vi "UNITEST MAIN v2.0.vi"() -> ()   [LabVIEW 2025] (continued)
        n1104 = call-poly "Enqueue Message.vi"("Priority Message? (F)"=TRUE, "Message"="Calculate Rotary", "Message Queue"=w1702) -> ("error out"=w1700:errorcluster, "dup Message Queue"=w1701:refnum<queue>)  [unwired: 7 in]
      }
      event "Clear List": Value Change {
        n1105 = event-data() -> ()  [unwired: 1 in, 1 out]
        n1106 = call-poly "Enqueue Message.vi"("Priority Message? (F)"=TRUE, "Message"="Clear List", "Message Queue"=w1707) -> ("error out"=w1705:errorcluster, "dup Message Queue"=w1706:refnum<queue>)  [unwired: 7 in]
      }
      event "Add to list": Value Change {
        n1107 = event-data() -> ()  [unwired: 1 in, 1 out]
        n1108 = call-poly "Enqueue Message.vi"("Priority Message? (F)"=TRUE, "Message"="Add to list", "Message Queue"=w1712) -> ("error out"=w1710:errorcluster, "dup Message Queue"=w1711:refnum<queue>)  [unwired: 7 in]
      }
      event "ClrLog": Value Change {
        n1109 = event-data() -> ()  [unwired: 1 in, 1 out]
        n1110 = call-poly "Enqueue Message.vi"("Priority Message? (F)"=TRUE, "Message"="ClrLog", "Message Queue"=w1717) -> ("error out"=w1715:errorcluster, "dup Message Queue"=w1716:refnum<queue>)  [unwired: 7 in]
      }
      event "Disable Axis Jog Soft Limits m": Value Change {
        n1111 = event-data() -> ()  [unwired: 1 in, 1 out]
        n1112 = call-poly "Enqueue Message.vi"("Priority Message? (F)"=TRUE, "Message"="Disable Axis Jog Soft Limits", "Message Queue"=w1722) -> ("error out"=w1720:errorcluster, "dup Message Queue"=w1721:refnum<queue>)  [unwired: 7 in]
      }
      event "Home Service": Value Change {
        n1113 = event-data() -> ()  [unwired: 1 in, 1 out]
        n1114 = call-poly "Enqueue Message.vi"("Priority Message? (F)"=TRUE, "Message"="Home Service", "Message Queue"=w1727) -> ("error out"=w1725:errorcluster, "dup Message Queue"=w1726:refnum<queue>)  [unwired: 7 in]
      }
      event "Edit Gain Constants": Value Change {
        n1115 = event-data() -> ()  [unwired: 1 in, 1 out]
        n1116 = call-poly "Enqueue Message.vi"("Priority Message? (F)"=TRUE, "Message"="Edit Gain Constants", "Message Queue"=w1732) -> ("error out"=w1730:errorcluster, "dup Message Queue"=w1731:refnum<queue>)  [unwired: 7 in]
      }
      event "Advanced Setting": Value Change {
        n1117 = event-data() -> ()  [unwired: 1 in, 1 out]
        n1118 = call-poly "Enqueue Message.vi"("Priority Message? (F)"=TRUE, "Message"="Advanced Setting", "Message Queue"=w1737) -> ("error out"=w1735:errorcluster, "dup Message Queue"=w1736:refnum<queue>)  [unwired: 7 in]
      }
      event "Password": Value Change {
        n1119 = event-data() -> ()  [unwired: 1 in, 1 out]
        n1120 = call-poly "Enqueue Message.vi"("Priority Message? (F)"=TRUE, "Message"="Password", "Message Queue"=w1742) -> ("error out"=w1740:errorcluster, "dup Message Queue"=w1741:refnum<queue>)  [unwired: 7 in]
      }
      event "Service About": Value Change {
        n1121 = event-data() -> ()  [unwired: 1 in, 1 out]
        n1122 = call-poly "Enqueue Message.vi"("Priority Message? (F)"=TRUE, "Message"="Service About", "Message Queue"=w1747) -> ("error out"=w1745:errorcluster, "dup Message Queue"=w1746:refnum<queue>)  [unwired: 7 in]
      }
      event "OPEN 1": Value Change {
        n1123 = event-data() -> ()  [unwired: 1 in, 1 out]
        n1124 = call-poly "Enqueue Message.vi"("Priority Message? (F)"=TRUE, "Message"="OPEN 1", "Message Queue"=w1752) -> ("error out"=w1750:errorcluster, "dup Message Queue"=w1751:refnum<queue>)  [unwired: 7 in]
      }
      event "OPEN 2": Value Change {
        n1125 = event-data() -> ()  [unwired: 1 in, 1 out]
        n1126 = call-poly "Enqueue Message.vi"("Priority Message? (F)"=TRUE, "Message"="OPEN 2", "Message Queue"=w1757) -> ("error out"=w1755:errorcluster, "dup Message Queue"=w1756:refnum<queue>)  [unwired: 7 in]
      }
      event "OPEN 3": Value Change {
        n1127 = event-data() -> ()  [unwired: 1 in, 1 out]
        n1128 = call-poly "Enqueue Message.vi"("Priority Message? (F)"=TRUE, "Message"="OPEN 3", "Message Queue"=w1762) -> ("error out"=w1760:errorcluster, "dup Message Queue"=w1761:refnum<queue>)  [unwired: 7 in]
      }
      event "OPEN 4": Value Change {
        n1129 = event-data() -> ()  [unwired: 1 in, 1 out]
        n1130 = call-poly "Enqueue Message.vi"("Priority Message? (F)"=TRUE, "Message"="OPEN 4", "Message Queue"=w1767) -> ("error out"=w1765:errorcluster, "dup Message Queue"=w1766:refnum<queue>)  [unwired: 7 in]
      }
      event "Refresh 2": Value Change {
        n1131 = event-data() -> ()  [unwired: 1 in, 1 out]
        n1132 = call-poly "Enqueue Message.vi"("Priority Message? (F)"=TRUE, "Message"="Refresh 2", "Message Queue"=w1772) -> ("error out"=w1770:errorcluster, "dup Message Queue"=w1771:refnum<queue>)  [unwired: 7 in]
      }
      event "Analysis Home new": Value Change {
        n1133 = event-data() -> ()  [unwired: 1 in, 1 out]
        n1134 = call-poly "Enqueue Message.vi"("Priority Message? (F)"=TRUE, "Message"="Analysis Home", "Message Queue"=w1777) -> ("error out"=w1775:errorcluster, "dup Message Queue"=w1776:refnum<queue>)  [unwired: 7 in]
      }
      event "Post Analysis": Value Change {
        n1135 = event-data() -> ()  [unwired: 1 in, 1 out]
        n1136 = call-poly "Enqueue Message.vi"("Priority Message? (F)"=TRUE, "Message"="Post Analysis", "Message Queue"=w1782) -> ("error out"=w1780:errorcluster, "dup Message Queue"=w1781:refnum<queue>)  [unwired: 7 in]
      }
      event "Scratch Mode": Value Change {
        n1137 = event-data() -> ()  [unwired: 1 in, 1 out]
        n1138 = call-poly "Enqueue Message.vi"("Priority Message? (F)"=TRUE, "Message"="Scratch Mode", "Message Queue"=w1787) -> ("error out"=w1785:errorcluster, "dup Message Queue"=w1786:refnum<queue>)  [unwired: 7 in]
      }
      event "Export": Value Change {
        n1139 = event-data() -> ()  [unwired: 1 in, 1 out]
        n1140 = call-poly "Enqueue Message.vi"("Priority Message? (F)"=TRUE, "Message"="Export", "Message Queue"=w1792) -> ("error out"=w1790:errorcluster, "dup Message Queue"=w1791:refnum<queue>)  [unwired: 7 in]
      }
      event "Traction Receipe Update Details": Value Change {
        n1141 = event-data() -> ()  [unwired: 1 in, 1 out]
        n1142 = call-poly "Enqueue Message.vi"("Priority Message? (F)"=TRUE, "Message"="Traction Receipe Update Details", "Message Queue"=w1797) -> ("error out"=w1795:errorcluster, "dup Message Queue"=w1796:refnum<queue>)  [unwired: 7 in]
      }
      event "Manual Write TRACTION": Value Change {
        n1143 = event-data() -> ()  [unwired: 1 in, 1 out]
        n1144 = call-poly "Enqueue Message.vi"("Priority Message? (F)"=TRUE, "Message"="Manual Write TRACTION", "Message Queue"=w1802) -> ("error out"=w1800:errorcluster, "dup Message Queue"=w1801:refnum<queue>)  [unwired: 7 in]
      }
      event "Manual Write Acquostic": Value Change {
        n1145 = event-data() -> ()  [unwired: 1 in, 1 out]
        n1146 = call-poly "Enqueue Message.vi"("Priority Message? (F)"=TRUE, "Message"="Manual Write ACQUOSTIC", "Message Queue"=w1807) -> ("error out"=w1805:errorcluster, "dup Message Queue"=w1806:refnum<queue>)  [unwired: 7 in]
      }
      event "Report": Value Change {
        n1147 = event-data() -> ()  [unwired: 1 in, 1 out]
        n1148 = call-poly "Enqueue Message.vi"("Priority Message? (F)"=TRUE, "Message"="Report", "Message Queue"=w1812) -> ("error out"=w1810:errorcluster, "dup Message Queue"=w1811:refnum<queue>)  [unwired: 7 in]
      }
      event "Acoustic Emission 3": Value Change {
        n1149 = event-data() -> ()  [unwired: 1 in, 1 out]
        n1150 = call-poly "Enqueue Message.vi"("Priority Message? (F)"=TRUE, "Message"="Acoustic Emission 3", "Message Queue"=w1817) -> ("error out"=w1815:errorcluster, "dup Message Queue"=w1816:refnum<queue>)  [unwired: 7 in]
      }
      event Application Instance Close {
        # "#CodeRecommended - When a project closes, all VIs within that project are aborted and leave memory. However, any code placed in this event frame is guaranteed to run to completion, so add any cleanup code that absolutely must happen here."
        n1151 = event-data() -> ()  [unwired: 1 in, 1 out]
      }
      event "EXIT": Value Change {
        n1152 = event-data() -> ()  [unwired: 1 in, 1 out]
        n1153 = call-poly "Enqueue Message.vi"("Priority Message? (F)"=TRUE, "Message"="Exit", "Message Queue"=w1825) -> ("error out"=w1824:errorcluster, "dup Message Queue"=w1823:refnum<queue>)  [unwired: 7 in]
      }
      event User Event {
        # "The Message Handling Loop processed an \"Exit\" message, which fired this event to stop the Event Handling Loop."
        n1154 = event-data() -> ()  [unwired: 1 in, 1 out]
      }
    }
    n1155 = call "LAB-IQ Error Handler - Event Handling Loop.vi"("error in (no error)"=w1435, "Message Queue"=w1433) -> ("dup error in"=w1432:errorcluster)  [unwired: 8 in, 1 out]
  }
  n1156 = timed-loop "Timed Loop" {
    shift-right: [w1838] -> _
    shift-left: w9 -> [w1839]
    tunnel: [w1832] -> w47
    tunnel: w35 -> [w1830]
    tunnel: w6 -> [w1829]
    tunnel: w10 -> [w1828]
    timing: w20 -> [_]
    timing-out: [_] -> w19
    stop <- w1837 stop-if-true
    # "Heave Motor  Handling Loop"
    n1157 = node-c288() -> ()  [unwired: 1 in, 1 out]
    n1158 = call "Dequeue Message.vi"("error in (no error)"=w1829, "Message Queue"=w1830) -> ("error out"=w1836:errorcluster, "Message Data"=w1834:variant, "Message"=w1835:string, "dup Message Queue"=w1833:refnum<queue>)  [unwired: 6 in]
    n1159 = case "Message Cases" shown="\"init\"" w1835 {
      selector: w1835 -> [_ _ _ _ _ w1934]
      tunnel: w1833 -> [w1854 w1870 _ w1922 w1933 _]
      tunnel: w1836 -> [w1851 w1868 w1914 w1925 w1927 _]
      tunnel: [w1852 w1871 w1908 w1915 w1929 w1935] -> w1831
      tunnel: w1839 -> [w1843 w1856 w1913 w1918 w1932 w1936]
      tunnel: [w1843 w1856 w1913 w1918 w1932 w1936] -> w1838
      tunnel: [_ _ _ _ TRUE _] -> w1837
      tunnel: w1834 -> [_ _ w1912 _ _ _]
      tunnel: w1828 -> [_ _ _ _ w1926 _]
      frame "init" {
        # "Initialize - All initialization work should take place in this message, since other loops can potentially enqueue messages that execute immediately after this one."
        n1160 = call "HEAVE WRITE FGV.vi"("Enum - Menu"=Heave_Write_enum."INIT", "error in (no error)"=w1851, "main ref"=w1843) -> ("error out"=w1850:errorcluster)  [unwired: 8 in]
        n1161 = call <vilib>:"Clear Errors.vi"("error in (no error)"=w1850) -> ("error out"=w1845:errorcluster)  [unwired: 5 in, 1 out]
        n1162 = call "Stall Data Flow.vim"("value in"=w1845, "milliseconds to wait"=u32 1000) -> ("value out"=w1848:errorcluster)  [unwired: 1 out]
        n1163 = call "Heave Init.vi"("error in (no error)"=w1848, "main ref"=w1843) -> ("error out"=w1846:errorcluster)  [unwired: 9 in]
        n1164 = call "HEAVE READ FGV.vi"("Enum - Menu"=Heave_Right_enum."INIT", "error in (no error)"=w1846, "main ref"=w1843) -> ("error out"=w1844:errorcluster)  [unwired: 6 in, 2 out]
        n1165 = call <vilib>:"Clear Errors.vi"("error in (no error)"=w1844) -> ("error out"=w1853:errorcluster)  [unwired: 5 in, 1 out]
        n1166 = call-poly "Enqueue Message.vi"("error in (no error)"=w1853, "Message"="Heave Main", "Message Queue"=w1854) -> ("error out"=w1852:errorcluster)  [unwired: 7 in, 1 out]
      }
      frame "Heave Main" {
        n1167 = Unbundle By Name(w1856) -> ("Heave AND Surge.Read Heave Temp"=w1864:refnum<vi>)
        n1168 = property on="Property Node" class="Bool (strict)"(reference=w1864) -> (reference out=w1862:refnum<vi>, error out=w1863:errorcluster, "Value"=w1861:bool)  [unwired: 1 in]
        n1169 = Close Reference(reference=w1862, error in (no error)=w1863) -> ()  [unwired: 1 out]
        n1170 = case shown="True" w1861 {
          tunnel: w1868 -> [w1894 w1899]
          tunnel: [w1894 w1898] -> w1859
          tunnel: w1856 -> [_ w1897]
          tunnel: [FALSE ("x < y?") w1896] -> w1857
          frame False {
          }
          frame True {
            n1171 = call "HEAVE READ FGV.vi"("Enum - Menu"=Heave_Right_enum."READ", "error in (no error)"=w1899, "main ref"=w1897) -> ("error out"=w1898:errorcluster, "x < y?"=w1896:bool)  [unwired: 6 in, 1 out]
          }
        }
        n1172 = case shown="True" w1857 {
          tunnel: w1856 -> [w1874 w1881]
          frame False {
            w1872 = TRUE ("PAUSE")
            w1873 = FALSE ("Value")
            n1173 = Unbundle By Name(w1874) -> ("Platform Settings.Heave COM Status"=w1880:refnum<vi>)
            n1174 = Unbundle By Name(w1874) -> ("Main Screen.Heave COM Status"=w1875:refnum<vi>)
            n1175 = property on="Property Node" class="Bool (strict)"(reference=w1880, "Value"=w1873) -> (reference out=w1878:refnum<vi>, error out=w1879:errorcluster)  [unwired: 1 in]
            n1176 = property on="Property Node" class="Bool (strict)"(reference=w1875, "Value"=w1873) -> (reference out=w1877:refnum<vi>, error out=w1876:errorcluster)  [unwired: 1 in]
            n1177 = Close Reference(reference=w1878, error in (no error)=w1879) -> ()  [unwired: 1 out]
            n1178 = Close Reference(reference=w1877, error in (no error)=w1876) -> ()  [unwired: 1 out]
            n1179 = call "ELAPSED TIMER VI FOR Sway Loop Connection.vi"("RESET"=w1872, "PAUSE"=w1872) -> ()  [unwired: 7 in, 3 out]
          }
          frame True {
            w1884 = FALSE ("PAUSE")
            n1180 = call "ELAPSED TIMER VI FOR Sway Loop Connection.vi"("TARGET"=2.0, "RESET"=w1884, "PAUSE"=w1884) -> ("ELAPSED INDICATION"=w1882:bool)  [unwired: 6 in, 2 out]
            n1181 = case shown="True" w1882 {
              tunnel: w1881 -> [_ w1885]
              frame False {
              }
              frame True {
                w1886 = TRUE ("Value")
                n1182 = Unbundle By Name(w1885) -> ("Main Screen.Heave COM Status"=w1887:refnum<vi>)
                n1183 = Unbundle By Name(w1885) -> ("Platform Settings.Heave COM Status"=w1892:refnum<vi>)
                n1184 = property on="Property Node" class="Bool (strict)"(reference=w1887, "Value"=w1886) -> (reference out=w1889:refnum<vi>, error out=w1888:errorcluster)  [unwired: 1 in]
                n1185 = property on="Property Node" class="Bool (strict)"(reference=w1892, "Value"=w1886) -> (reference out=w1890:refnum<vi>, error out=w1891:errorcluster)  [unwired: 1 in]
                n1186 = Close Reference(reference=w1889, error in (no error)=w1888) -> ()  [unwired: 1 out]
                n1187 = Close Reference(reference=w1890, error in (no error)=w1891) -> ()  [unwired: 1 out]
              }
            }
          }
        }
        n1188 = call "Heave Reinitial.vi"("error in (no error)"=w1859, "Data Cluster"=w1856) -> ("error out"=w1858:errorcluster)  [unwired: 9 in]
        n1189 = Unbundle By Name(w1856) -> ("Main Home Screen.EXIT"=w1869:refnum<vi>)
        n1190 = property on="Property Node" class="Bool (strict)"(reference=w1869) -> (reference out=w1866:refnum<vi>, error out=w1867:errorcluster, "Value"=w1865:bool)  [unwired: 1 in]
        n1191 = call <vilib>:"Clear Errors.vi"("error in (no error)"=w1858) -> ("error out"=w1860:errorcluster)  [unwired: 5 in, 1 out]
        n1192 = Close Reference(reference=w1866, error in (no error)=w1867) -> ()  [unwired: 1 out]
        n1193 = case shown="False" w1865 {
          tunnel: [w1902 w1906] -> w1871
          tunnel: w1870 -> [w1901 w1905]
          tunnel: w1860 -> [w1900 w1904]
          frame True {
            n1194 = call-poly "Enqueue Message.vi"("error in (no error)"=w1900, "Message"="Confirm Quit", "Message Queue"=w1901) -> ("error out"=w1902:errorcluster)  [unwired: 7 in, 1 out]
          }
          frame False {
            n1195 = call-poly "Enqueue Message.vi"("error in (no error)"=w1904, "Message"="Heave Main", "Message Queue"=w1905) -> ("error out"=w1906:errorcluster)  [unwired: 7 in, 1 out]
          }
        }
      }
      frame "Error" {
        # "#CodeRecommended - If you ever change the name of this \"Error\" message, you'll need to update the name in the Check Loop Error.vi as well."
        # "#CodeRecommended - Consider creating a system for logging errors in some way. These errors are for notification purposes only. Handling of specific errors should be performed in the message frames that generated the error."
        # "Error - Display an error dialog. This message is sent by the \"Error Handler\" VIs at the end of other loops in this application."
        n1196 = Variant To Data(error in=w1914, type=errorcluster {"status"=FALSE, "code"=0, "source"=""} ("error constant"), Variant=w1912) -> (data=w1910:errorcluster, error out=w1909:errorcluster)
        n1197 = call <vilib>:"Simple Error Handler.vi"("error in (no error)"=w1910) -> ()  [unwired: 4 in, 5 out]
        n1198 = Merge Errors(w1909) -> (w1908:errorcluster)
      }
      frame "Confirm Quit" {
        # "#CodeNeeded - If you want to provide an \"Are you sure\" dialog (or some other notification) before the application exits, place that code here. This message is typically sent from a Panel Close? event."
        # "Confirm Quit - Message that can confirm whether or not the user wants to exit the application."
        n1199 = call-poly "Enqueue Message.vi"("Priority Message? (F)"=TRUE, "error in (no error)"=w1925, "Message"="Exit", "Message Queue"=w1922) -> ("error out"=w1923:errorcluster)  [unwired: 6 in, 1 out]
        n1200 = Merge Errors(w1923) -> (w1924:errorcluster)
        n1201 = call <vilib>:"Clear Errors.vi"("error in (no error)"=w1924) -> ("error out"=w1916:errorcluster)  [unwired: 5 in, 1 out]
        n1202 = call "HEAVE WRITE FGV.vi"("Enum - Menu"=Heave_Write_enum."CLOSE", "error in (no error)"=w1916, "main ref"=w1918) -> ("error out"=w1919:errorcluster)  [unwired: 8 in]
        n1203 = call <vilib>:"Clear Errors.vi"("error in (no error)"=w1919) -> ("error out"=w1915:errorcluster)  [unwired: 5 in, 1 out]
      }
      frame "Exit" {
        # "Stop the VI"
        # "Release the message queue reference"
        # "#CodeNeeded - Add any required cleanup code here. Note that if 'Exit' was called as a result of an error, an error dialog will be displayed. Add any custom error handling for an 'Exit' condition here as well."
        # "Exit - Exit the application."
        n1204 = call "Fire User Event - Stop.vi"("User Event - Stop"=w1926) -> ("error out"=w1928:errorcluster)  [unwired: 10 in]
        n1205 = Release Queue(queue=w1933, error in (no error)=w1927) -> (error out=w1930:errorcluster)  [unwired: 1 in, 2 out]
        n1206 = Merge Errors(w1928, w1930) -> (w1929:errorcluster)
      }
      frame Default {
        # "'Default' case only runs if there is a message that isn't defined in any of the other cases.  Output a programming error."
        n1207 = xnode ("Error Ring")("parameter 0"=w1934) -> ("error out"=w1935:errorcluster)
      }
    }
    n1208 = call "LAB-IQ Error Handler - Message Handling Loop.vi"("error in (no error)"=w1831, "Message Queue"=w1833) -> ("dup error in"=w1832:errorcluster)  [unwired: 8 in, 1 out]
    n1209 = node-c288() -> ()  [unwired: 1 in, 1 out]
  }
  n1210 = while {
    tunnel: w78 -> [w1947]
    shift-right: [w1954] -> _
    shift-left: w9 -> [w1955]
    tunnel: w10 -> [w1952]
    tunnel: w71 -> [w1951]
    tunnel: [w1945] -> w79
    stop <- w1953 stop-if-true
    # "Message Handling Loop"
    n1211 = call "Dequeue Message.vi"("error in (no error)"=w1951, "Message Queue"=w1947) -> ("error out"=w1950:errorcluster, "Message Data"=w1948:variant, "Message"=w1949:string, "dup Message Queue"=w1946:refnum<queue>)  [unwired: 6 in]
    n1212 = case "Message Cases" shown="\"SNext\"" w1949 {
      selector: w1949 -> [_ _ _ _ _ _ _ _ _ _ _ _ _ _ _ _ _ _ _ _ _ _ _ _ _ _ _ _ _ _ _ _ _ _ _ _ _ _ _ _ _ _ _ _ _ _ _ _ _ _ _ _ _ _ _ _ _ _ _ _ _ _ _ _ _ _ _ _ _ _ _ _ _ _ _ _ _ _ _ _ w3342]
      tunnel: w1946 -> [_ w2004 _ _ _ _ _ _ _ _ _ _ _ _ _ _ _ _ _ _ _ _ _ _ _ _ _ _ _ _ _ _ _ _ _ _ _ _ _ _ _ _ _ _ _ _ _ _ _ _ _ _ _ _ _ _ _ _ _ _ _ _ _ _ _ _ _ _ _ _ _ _ _ _ _ _ _ _ w3330 w3341 _]
      tunnel: w1950 -> [w1958 w2006 w2010 w2019 w2040 w2057 w2074 w2091 w2112 w2125 w2130 w2134 w2141 w2146 w2211 w2237 w2263 w2298 w2314 w2366 w2370 w2373 w2376 w2383 w2459 w2471 w2488 w2499 w2526 w2537 w2548 w2559 w2570 w2581 w2592 w2603 w2615 w2626 w2637 w2648 w2657 w2668 w2678 w2689 w2696 w2726 w2767 w2773 w2805 w2813 w2816 w2824 w2836 w2845 w2865 w2879 w2889 w2899 w2901 w2916 w2929 w2946 w2963 w2999 w3007 w3066 w3090 w3100 w3141 w3184 w3227 w3263 w3270 w3289 w3295 w3303 w3319 w3326 w3333 w3334 _]
      tunnel: [w1957 w1973 w2015 w2020 w2035 w2052 w2069 w2086 w2107 w2117 w2128 w2132 w2139 w2150 w2207 w2233 w2259 w2299 w2315 w2330 w2369 w2372 w2375 w2382 w2453 w2470 w2489 w2512 w2528 w2539 w2550 w2561 w2572 w2583 w2594 w2605 w2616 w2627 w2638 w2649 w2659 w2669 w2679 w2690 w2695 w2725 w2746 w2778 w2786 w2812 w2815 w2823 w2830 w2840 w2858 w2878 w2889 w2899 w2907 w2915 w2928 w2945 w2962 w2998 w3006 w3066 w3090 w3097 w3138 w3181 w3224 w3264 w3270 w3283 w3293 w3302 w3317 w3320 w3332 w3337 w3343] -> w1944
      tunnel: w1955 -> [w1956 w1960 w2011 w2018 w2026 w2043 w2060 w2077 w2095 w2115 w2127 w2131 w2137 w2145 w2209 w2235 w2261 w2286 w2301 w2317 w2368 w2371 w2374 w2377 w2452 w2469 w2482 w2496 w2524 w2535 w2546 w2557 w2568 w2579 w2590 w2601 w2613 w2624 w2635 w2646 w2656 w2667 w2677 w2688 w2694 w2724 w2745 w2771 w2784 w2811 w2814 w2818 w2829 w2838 w2860 w2877 w2881 w2891 w2900 w2914 w2918 w2931 w2949 w2965 w3001 w3058 w3081 w3093 w3134 w3177 w3220 w3262 w3265 w3282 w3292 w3297 w3316 w3325 w3327 w3340 w3344]
      tunnel: [w1956 w1960 w2011 w2018 w2026 w2043 w2060 w2077 w2095 w2115 w2127 w2131 w2137 w2145 w2209 w2235 w2261 w2286 w2301 w2317 w2368 w2371 w2374 w2377 w2452 w2469 w2482 w2496 w2524 w2535 w2546 w2557 w2568 w2579 w2590 w2601 w2613 w2624 w2635 w2646 w2656 w2667 w2677 w2688 w2694 w2724 w2745 w2771 w2784 w2811 w2814 w2818 w2829 w2838 w2860 w2877 w2881 w2891 w2900 w2914 w2918 w2931 w2949 w2965 w3001 w3058 w3081 w3093 w3134 w3177 w3220 w3262 w3265 w3282 w3292 w3297 w3316 w3325 w3327 w3340 w3344] -> w1954
      tunnel: [_ _ _ _ _ _ _ _ _ _ _ _ _ _ _ _ _ _ _ _ _ _ _ _ _ _ _ _ _ _ _ _ _ _ _ _ _ _ _ _ _ _ _ _ _ _ _ _ _ _ _ _ _ _ _ _ _ _ _ _ _ _ _ _ _ _ _ _ _ _ _ _ _ _ _ _ _ _ _ TRUE _] -> w1953
      tunnel: w1948 -> [_ _ _ _ _ _ _ _ _ _ _ _ _ _ _ _ _ _ _ _ _ _ _ _ _ _ _ _ _ _ _ _ _ _ _ _ _ _ _ _ _ _ _ _ _ _ _ _ _ _ _ _ _ _ _ _ _ _ _ _ _ _ _ _ _ _ _ _ _ _ _ _ _ _ _ _ _ w3324 _ _ _]
      tunnel: w1952 -> [_ _ _ _ _ _ _ _ _ _ _ _ _ _ _ _ _ _ _ _ _ _ _ _ _ _ _ _ _ _ _ _ _ _ _ _ _ _ _ _ _ _ _ _ _ _ _ _ _ _ _ _ _ _ _ _ _ _ _ _ _ _ _ _ _ _ _ _ _ _ _ _ _ _ _ _ _ _ _ w3336 _]
      frame "Timeout" {
        n1213 = call "Time Out Loop.vi"("error in (no error)"=w1958, "Data Cluster"=w1956) -> ("error out"=w1957:errorcluster)  [unwired: 9 in]
      }
      frame "init" {
        # "Initialize - All initialization work should take place in this message, since other loops can potentially enqueue messages that execute immediately after this one."
        n1214 = Unbundle By Name(w1960) -> ("Loading.Warning"=w1963:refnum<vi>)
        n1215 = property class="TabCtl (strict)"(reference=w1963, "Visible"=FALSE) -> (reference out=w1961:refnum<vi>, error out=w1962:errorcluster)  [unwired: 1 in]
        n1216 = call-poly "Enqueue Message.vi"("error in (no error)"=w2006, "Message"="Init Other Loop", "Message Queue"=w2004) -> ("error out"=w2007:errorcluster)  [unwired: 7 in, 1 out]
        n1217 = Close Reference(reference=w1961, error in (no error)=w1962) -> ()  [unwired: 1 out]
        n1218 = Unbundle By Name(w1960) -> ("Loading.SSP 0.3"=w1992:refnum<vi>)
        n1219 = Unbundle By Name(w1960) -> ("Loading.SSP 0.5"=w1989:refnum<vi>)
        n1220 = Unbundle By Name(w1960) -> ("Loading.SSP 0.75"=w1984:refnum<vi>)
        n1221 = Unbundle By Name(w1960) -> ("Loading.Communication is established"=w1979:refnum<vi>)
        n1222 = Unbundle By Name(w1960) -> ("Loading Com Port.Load Cell Temp"=w1998:refnum<vi>)
        n1223 = Unbundle By Name(w1960) -> ("Motion Module.Set WTD"=w1972:refnum<vi>)
        n1224 = call "Read Config Unitest.vi"("error in (no error)"=w2007, "main ref"=w1960) -> ("error out"=w2002:errorcluster)  [unwired: 9 in]
        n1225 = Unbundle By Name(w1960) -> ("Motion Module.Wear Track Diameter"=w1966:refnum<vi>)
        n1226 = Unbundle By Name(w1960) -> ("PID.Ramp"=w1976:refnum<vi>)
        n1227 = call "Encrypt file path creation.vi"("error in (no error)"=w2002) -> ("error out"=w2001:errorcluster, "File Path"=w2000:path)  [unwired: 9 in]
        n1228 = property on="Property Node" class="Bool (strict)"(reference=w1998, "Value"=FALSE) -> (reference out=w1996:refnum<vi>, error out=w1997:errorcluster)  [unwired: 1 in]
        n1229 = property on="Property Node" class="Bool (strict)"(reference=w1989, "Visible"=FALSE) -> (reference out=w1987:refnum<vi>, error out=w1988:errorcluster)  [unwired: 1 in]
        n1230 = property on="Property Node" class="Bool (strict)"(reference=w1992, "Visible"=FALSE) -> (reference out=w1994:refnum<vi>, error out=w1993:errorcluster)  [unwired: 1 in]
        n1231 = property on="Property Node" class="Bool (strict)"(reference=w1984, "Visible"=FALSE) -> (reference out=w1986:refnum<vi>, error out=w1985:errorcluster)  [unwired: 1 in]
        n1232 = property on="Property Node" class="Bool (strict)"(reference=w1976, "Value"=FALSE) -> (reference out=w1978:refnum<vi>, error out=w1977:errorcluster)  [unwired: 1 in]
        n1233 = property on="Property Node" class="DigNum (strict)"(reference=w1966, "Value"=0.0) -> (reference out=w1965:refnum<vi>, error out=w1967:errorcluster)  [unwired: 1 in]
        n1234 = property on="Property Node" class="Bool (strict)"(reference=w1972, "Visible"=FALSE, "DisabledEnum"=T31."Disabled and Grayed Out" ("Disabled")) -> (reference out=w1969:refnum<vi>, error out=w1971:errorcluster)  [unwired: 1 in]
        n1235 = property on="Property Node" class="Bool (strict)"(reference=w1979, "Visible"=FALSE ("Value")) -> (reference out=w1981:refnum<vi>, error out=w1980:errorcluster)  [unwired: 1 in]
        n1236 = call "DATA ENCRYPT STRING FILE WRITE.vi"("file path (dialog if empty)"=w2000, "error in (no error)"=w2001, "User Action"="System Booted", "main ref"=w1960) -> ("error out"=w2003:errorcluster)  [unwired: 5 in, 1 out]
        n1237 = Close Reference(reference=w1987, error in (no error)=w1988) -> ()  [unwired: 1 out]
        n1238 = Close Reference(reference=w1994, error in (no error)=w1993) -> ()  [unwired: 1 out]
        n1239 = Close Reference(reference=w1986, error in (no error)=w1985) -> ()  [unwired: 1 out]
        n1240 = Close Reference(reference=w1978, error in (no error)=w1977) -> ()  [unwired: 1 out]
        n1241 = Close Reference(reference=w1996, error in (no error)=w1997) -> ()  [unwired: 1 out]
        n1242 = Close Reference(reference=w1965, error in (no error)=w1967) -> ()  [unwired: 1 out]
        n1243 = Close Reference(reference=w1969, error in (no error)=w1971) -> ()  [unwired: 1 out]
        n1244 = Close Reference(reference=w1981, error in (no error)=w1980) -> ()  [unwired: 1 out]
        n1245 = call "Reinitial Parameter After Test.vi"("error in (no error)"=w2003, "main ref"=w1960) -> ("error out"=w1973:errorcluster)  [unwired: 9 in]
        n1246 = local write "HEAVE ENABLE"(FALSE ("HEAVE ENABLE")) -> ()
      }
      frame "Init Other Loop" {
        n1247 = Unbundle By Name(w2011) -> ("Loading.com 3"=w2014:refnum<vi>)
        n1248 = property on="Property Node" class="Bool (strict)"(reference=w2014, error in=w2010, "Value"=TRUE) -> (reference out=w2012:refnum<vi>, error out=w2013:errorcluster)
        n1249 = Close Reference(reference=w2012, error in (no error)=w2013) -> (error out=w2009:errorcluster)
        n1250 = call "SET LOAD PARAMETERS.vi"("error in (no error)"=w2009, "main ref"=w2011) -> ("error out"=w2015:errorcluster)  [unwired: 9 in]
      }
      frame "Service Save" {
        n1251 = call "Write Config Unitest.vi"("error in (no error)"=w2019, "main ref"=w2018) -> ("error out"=w2024:errorcluster)  [unwired: 9 in]
        n1252 = call "Stall Data Flow.vim"("value in"=w2024, "milliseconds to wait"=u32 2000) -> ("value out"=w2023:errorcluster)  [unwired: 1 out]
        n1253 = call "Read Config Unitest.vi"("error in (no error)"=w2023, "main ref"=w2018) -> ("error out"=w2021:errorcluster)  [unwired: 9 in]
        n1254 = local write "SAVE  2"(FALSE ("SAVE  2")) -> ()
        n1255 = call "DATA ENCRYPT STRING FILE WRITE.vi"("error in (no error)"=w2021, "User Action"="Service Parameter Saved", "main ref"=w2018) -> ("error out"=w2020:errorcluster)  [unwired: 6 in, 1 out]
      }
      frame "HOME" {
        n1256 = call "DATA ENCRYPT STRING FILE WRITE.vi"("error in (no error)"=w2040, "User Action"="User Pressed Home", "main ref"=w2026) -> ("error out"=w2036:errorcluster)  [unwired: 6 in, 1 out]
        n1257 = Unbundle By Name(w2026) -> ("Main Home Screen.MainPage"=w2031:refnum<vi>)
        n1258 = Unbundle By Name(w2026) -> ("Main Home Screen.Home"=w2039:refnum<vi>)
        n1259 = Unbundle By Name(w2026) -> ("Main Home Screen.GUI"=w2029:refnum<vi>)
        n1260 = property on="Property Node" class="Bool (strict)"(reference=w2039, error in=w2036, "Value"=FALSE) -> (reference out=w2037:refnum<vi>, error out=w2038:errorcluster)
        n1261 = property on="Property Node" class="TabCtl (strict)"(reference=w2031, "Value"=T16."HOME") -> (reference out=w2033:refnum<vi>, error out=w2032:errorcluster)  [unwired: 1 in]
        n1262 = property on="Property Node" class="TabCtl (strict)"(reference=w2029, "Value"=T15."Setup") -> (reference out=w2027:refnum<vi>, error out=w2028:errorcluster)  [unwired: 1 in]
        n1263 = Close Reference(reference=w2037, error in (no error)=w2038) -> (error out=w2035:errorcluster)
        n1264 = Close Reference(reference=w2033, error in (no error)=w2032) -> ()  [unwired: 1 out]
        n1265 = Close Reference(reference=w2027, error in (no error)=w2028) -> ()  [unwired: 1 out]
      }
      frame "Platform Setting" {
        n1266 = call "DATA ENCRYPT STRING FILE WRITE.vi"("error in (no error)"=w2057, "User Action"="User Pressed Platform Setting", "main ref"=w2043) -> ("error out"=w2053:errorcluster)  [unwired: 6 in, 1 out]
        n1267 = Unbundle By Name(w2043) -> ("Main Home Screen.Platform Settings"=w2056:refnum<vi>)
        n1268 = Unbundle By Name(w2043) -> ("Main Home Screen.MainPage"=w2048:refnum<vi>)
        n1269 = Unbundle By Name(w2043) -> ("Main Home Screen.GUI"=w2046:refnum<vi>)
        n1270 = property on="Property Node" class="TabCtl (strict)"(reference=w2048, "Value"=T16."PlatformSetting") -> (reference out=w2050:refnum<vi>, error out=w2049:errorcluster)  [unwired: 1 in]
        n1271 = property on="Property Node" class="TabCtl (strict)"(reference=w2046, "Value"=T15."Setup") -> (reference out=w2044:refnum<vi>, error out=w2045:errorcluster)  [unwired: 1 in]
        n1272 = property on="Property Node" class="Bool (strict)"(reference=w2056, error in=w2053, "Value"=FALSE) -> (reference out=w2054:refnum<vi>, error out=w2055:errorcluster)
        n1273 = Close Reference(reference=w2050, error in (no error)=w2049) -> ()  [unwired: 1 out]
        n1274 = Close Reference(reference=w2044, error in (no error)=w2045) -> ()  [unwired: 1 out]
        n1275 = Close Reference(reference=w2054, error in (no error)=w2055) -> (error out=w2052:errorcluster)
      }
      frame "Configure" {
        n1276 = call "DATA ENCRYPT STRING FILE WRITE.vi"("error in (no error)"=w2074, "User Action"="User Pressed Configure", "main ref"=w2060) -> ("error out"=w2070:errorcluster)  [unwired: 6 in, 1 out]
        n1277 = Unbundle By Name(w2060) -> ("Main Home Screen.Configure"=w2073:refnum<vi>)
        n1278 = Unbundle By Name(w2060) -> ("Main Home Screen.MainPage"=w2065:refnum<vi>)
        n1279 = Unbundle By Name(w2060) -> ("Main Home Screen.GUI"=w2063:refnum<vi>)
        n1280 = property on="Property Node" class="Bool (strict)"(reference=w2073, error in=w2070, "Value"=FALSE) -> (reference out=w2071:refnum<vi>, error out=w2072:errorcluster)
        n1281 = property on="Property Node" class="TabCtl (strict)"(reference=w2065, "Value"=T16."Details") -> (reference out=w2067:refnum<vi>, error out=w2066:errorcluster)  [unwired: 1 in]
        n1282 = property on="Property Node" class="TabCtl (strict)"(reference=w2063, "Value"=T15."Setup") -> (reference out=w2061:refnum<vi>, error out=w2062:errorcluster)  [unwired: 1 in]
        n1283 = Close Reference(reference=w2071, error in (no error)=w2072) -> (error out=w2069:errorcluster)
        n1284 = Close Reference(reference=w2067, error in (no error)=w2066) -> ()  [unwired: 1 out]
        n1285 = Close Reference(reference=w2061, error in (no error)=w2062) -> ()  [unwired: 1 out]
      }
      frame "Analysis" {
        n1286 = call "DATA ENCRYPT STRING FILE WRITE.vi"("error in (no error)"=w2091, "User Action"="User Pressed Analysis", "main ref"=w2077) -> ("error out"=w2087:errorcluster)  [unwired: 6 in, 1 out]
        n1287 = Unbundle By Name(w2077) -> ("Main Home Screen.MainPage"=w2082:refnum<vi>)
        n1288 = Unbundle By Name(w2077) -> ("Main Home Screen.Analysis"=w2090:refnum<vi>)
        n1289 = Unbundle By Name(w2077) -> ("Main Home Screen.GUI"=w2080:refnum<vi>)
        n1290 = property on="Property Node" class="Bool (strict)"(reference=w2090, error in=w2087, "Value"=FALSE) -> (reference out=w2088:refnum<vi>, error out=w2089:errorcluster)
        n1291 = property on="Property Node" class="TabCtl (strict)"(reference=w2082, "Value"=T16."Analysis") -> (reference out=w2084:refnum<vi>, error out=w2083:errorcluster)  [unwired: 1 in]
        n1292 = property on="Property Node" class="TabCtl (strict)"(reference=w2080, "Value"=T15."Setup") -> (reference out=w2078:refnum<vi>, error out=w2079:errorcluster)  [unwired: 1 in]
        n1293 = Close Reference(reference=w2088, error in (no error)=w2089) -> (error out=w2086:errorcluster)
        n1294 = Close Reference(reference=w2084, error in (no error)=w2083) -> ()  [unwired: 1 out]
        n1295 = Close Reference(reference=w2078, error in (no error)=w2079) -> ()  [unwired: 1 out]
      }
      frame "service 2" {
        n1296 = call "DATA ENCRYPT STRING FILE WRITE.vi"("error in (no error)"=w2112, "User Action"="User Pressed service", "main ref"=w2095) -> ("error out"=w2108:errorcluster)  [unwired: 6 in, 1 out]
        n1297 = Unbundle By Name(w2095) -> ("Main Screen.Main Screen Tab"=w2096:refnum<vi>)
        n1298 = Unbundle By Name(w2095) -> ("Main Home Screen.MainPage"=w2103:refnum<vi>)
        n1299 = Unbundle By Name(w2095) -> ("Main Home Screen.Analysis"=w2111:refnum<vi>)
        n1300 = Unbundle By Name(w2095) -> ("Main Home Screen.GUI"=w2101:refnum<vi>)
        n1301 = property on="Property Node" class="Bool (strict)"(reference=w2111, error in=w2108, "Value"=FALSE) -> (reference out=w2109:refnum<vi>, error out=w2110:errorcluster)
        n1302 = property on="Property Node" class="TabCtl (strict)"(reference=w2103, "Value"=T16."HOME") -> (reference out=w2105:refnum<vi>, error out=w2104:errorcluster)  [unwired: 1 in]
        n1303 = property on="Property Node" class="TabCtl (strict)"(reference=w2101, "Value"=T15."Begin") -> (reference out=w2099:refnum<vi>, error out=w2100:errorcluster)  [unwired: 1 in]
        n1304 = property on="Property Node" class="TabCtl (strict)"(reference=w2096, "Value"=T19."About") -> (reference out=w2093:refnum<vi>, error out=w2097:errorcluster)  [unwired: 1 in]
        n1305 = Close Reference(reference=w2109, error in (no error)=w2110) -> (error out=w2107:errorcluster)
        n1306 = Close Reference(reference=w2105, error in (no error)=w2104) -> ()  [unwired: 1 out]
        n1307 = Close Reference(reference=w2099, error in (no error)=w2100) -> ()  [unwired: 1 out]
        n1308 = Close Reference(reference=w2093, error in (no error)=w2097) -> ()  [unwired: 1 out]
      }
      frame "Auto" {
        n1309 = call "DATA ENCRYPT STRING FILE WRITE.vi"("error in (no error)"=w2125, "User Action"="User Pressed Auto File Name", "main ref"=w2115) -> ("error out"=w2122:errorcluster)  [unwired: 6 in, 1 out]
        n1310 = Get Date/Time In Seconds() -> (seconds since 1Jan1904=w2123:timestamp)
        n1311 = Format Into String(format string="%<%I_%M_%S_%p_%d_%B_%Y>T", error in=w2122, w2123) -> (resulting string=w2116:string, error out=w2118:errorcluster)  [unwired: 1 in]
        n1312 = local write "Auto"(FALSE ("Auto")) -> ()
        n1313 = Unbundle By Name(w2115) -> ("Config Screen.FILE"=w2121:refnum<vi>)
        n1314 = property on="Property Node" class="Str"(reference=w2121, error in=w2118, "Value"=w2116) -> (reference out=w2119:refnum<vi>, error out=w2120:errorcluster)
        n1315 = Close Reference(reference=w2119, error in (no error)=w2120) -> (error out=w2117:errorcluster)
      }
      frame "Select Load Head" {
        n1316 = call "Reinitial Parameter.vi"("error in (no error)"=w2130, "Data Cluster"=w2127) -> ("error out"=w2129:errorcluster)  [unwired: 9 in]
        n1317 = call "FILE NAME RECHECK.vi"("error in (no error)"=w2129, "main ref"=w2127) -> ("error out"=w2128:errorcluster)  [unwired: 9 in]
      }
      frame "com 3" {
        n1318 = call "DATA ENCRYPT STRING FILE WRITE.vi"("error in (no error)"=w2134, "User Action"="User Pressed Check Load Communication", "main ref"=w2131) -> ("error out"=w2133:errorcluster)  [unwired: 6 in, 1 out]
        n1319 = call "SET LOAD PARAMETERS.vi"("error in (no error)"=w2133, "main ref"=w2131) -> ("error out"=w2132:errorcluster)  [unwired: 9 in]
      }
      frame "ZeroAll" {
        n1320 = call "DATA ENCRYPT STRING FILE WRITE.vi"("error in (no error)"=w2141, "User Action"="User Pressed Zero All", "main ref"=w2137) -> ("error out"=w2140:errorcluster)  [unwired: 6 in, 1 out]
        n1321 = local write "ZeroAll"(FALSE ("ZeroAll")) -> ()
        n1322 = call "LOAD CELL FGV MAIN.vi"("Enum"=T32."ZEROALL", "error in (no error)"=w2140, "main ref"=w2137) -> ("error IO"=w2139:errorcluster)  [unwired: 8 in]
      }
      frame "Loading Mode" {
        n1323 = Unbundle By Name(w2145) -> ("Loading.Loading Mode"=w2147:refnum<vi>)
        n1324 = property on="Property Node" class="Ring (strict)"(reference=w2147, error in=w2146) -> (reference out=w2149:refnum<vi>, error out=w2148:errorcluster, "Value"=w2143:u16)
        n1325 = Close Reference(reference=w2149, error in (no error)=w2148) -> (error out=w2144:errorcluster)
        n1326 = case shown="1" w2143 {
          tunnel: [w2164 w2181 w2193 w2205] -> w2150
          tunnel: w2145 -> [w2151 w2167 w2185 w2197]
          tunnel: w2144 -> [w2165 w2180 w2192 w2204]
          frame 0, Default {
            n1327 = Unbundle By Name(w2151) -> ("Loading.Enter the Loading Rate (N/min)"=w2158:refnum<vi>)
            n1328 = Unbundle By Name(w2151) -> ("Loading.Load Selection"=w2161:refnum<vi>)
            n1329 = Unbundle By Name(w2151) -> ("Loading.Enter the Final Load (N)"=w2153:refnum<vi>)
            n1330 = property on="Property Node" class="TabCtl (strict)"(reference=w2161, "Value"=T17."Constant") -> (reference out=w2163:refnum<vi>, error out=w2162:errorcluster)  [unwired: 1 in]
            n1331 = property on="Property Node" class="DigNum (strict)"(reference=w2158, "DisabledEnum"=T31."Disabled and Grayed Out" ("Disabled")) -> (reference out=w2157:refnum<vi>, error out=w2159:errorcluster)  [unwired: 1 in]
            n1332 = property on="Property Node" class="DigNum (strict)"(reference=w2153, "DisabledEnum"=T31."Disabled and Grayed Out" ("Disabled")) -> (reference out=w2154:refnum<vi>, error out=w2152:errorcluster)  [unwired: 1 in]
            n1333 = call "DATA ENCRYPT STRING FILE WRITE.vi"("error in (no error)"=w2165, "User Action"="User selected Constant Mode", "main ref"=w2151) -> ("error out"=w2164:errorcluster)  [unwired: 6 in, 1 out]
            n1334 = Close Reference(reference=w2163, error in (no error)=w2162) -> ()  [unwired: 1 out]
            n1335 = Close Reference(reference=w2157, error in (no error)=w2159) -> ()  [unwired: 1 out]
            n1336 = Close Reference(reference=w2154, error in (no error)=w2152) -> ()  [unwired: 1 out]
          }
          frame 1 {
            n1337 = Unbundle By Name(w2167) -> ("Loading.Enter the Loading Rate (N/min)"=w2178:refnum<vi>)
            n1338 = Unbundle By Name(w2167) -> ("Loading.Enter the Final Load (N)"=w2173:refnum<vi>)
            n1339 = Unbundle By Name(w2167) -> ("Loading.Load Selection"=w2169:refnum<vi>)
            n1340 = property on="Property Node" class="TabCtl (strict)"(reference=w2169, "Value"=T17."Constant") -> (reference out=w2171:refnum<vi>, error out=w2170:errorcluster)  [unwired: 1 in]
            n1341 = property on="Property Node" class="DigNum (strict)"(reference=w2178, "DisabledEnum"=T31."Enabled" ("Disabled")) -> (reference out=w2177:refnum<vi>, error out=w2179:errorcluster)  [unwired: 1 in]
            n1342 = property on="Property Node" class="DigNum (strict)"(reference=w2173, "DisabledEnum"=T31."Enabled" ("Disabled")) -> (reference out=w2174:refnum<vi>, error out=w2172:errorcluster)  [unwired: 1 in]
            n1343 = call "DATA ENCRYPT STRING FILE WRITE.vi"("error in (no error)"=w2180, "User Action"="User selected Ramp Mode", "main ref"=w2167) -> ("error out"=w2181:errorcluster)  [unwired: 6 in, 1 out]
            n1344 = Close Reference(reference=w2171, error in (no error)=w2170) -> ()  [unwired: 1 out]
            n1345 = Close Reference(reference=w2177, error in (no error)=w2179) -> ()  [unwired: 1 out]
            n1346 = Close Reference(reference=w2174, error in (no error)=w2172) -> ()  [unwired: 1 out]
          }
          frame 2 {
            n1347 = Unbundle By Name(w2185) -> ("Loading.Load Selection"=w2189:refnum<vi>)
            n1348 = Unbundle By Name(w2185) -> ("Loading.Warning 2"=w2187:refnum<vi>)
            n1349 = property on="Property Node" class="TabCtl (strict)"(reference=w2189, "Value"=T17."Step") -> (reference out=w2191:refnum<vi>, error out=w2190:errorcluster)  [unwired: 1 in]
            n1350 = property on="Property Node" class="Bool (strict)"(reference=w2187, "Visible"=FALSE) -> (reference out=w2183:refnum<vi>, error out=w2186:errorcluster)  [unwired: 1 in]
            n1351 = call "DATA ENCRYPT STRING FILE WRITE.vi"("error in (no error)"=w2192, "User Action"="User selected Step Mode", "main ref"=w2185) -> ("error out"=w2193:errorcluster)  [unwired: 6 in, 1 out]
            n1352 = Close Reference(reference=w2191, error in (no error)=w2190) -> ()  [unwired: 1 out]
            n1353 = Close Reference(reference=w2183, error in (no error)=w2186) -> ()  [unwired: 1 out]
          }
          frame 3 {
            n1354 = Unbundle By Name(w2197) -> ("Loading.Load Selection"=w2201:refnum<vi>)
            n1355 = Unbundle By Name(w2197) -> ("Loading.Warning 2"=w2199:refnum<vi>)
            n1356 = property on="Property Node" class="TabCtl (strict)"(reference=w2201, "Value"=T17."Indentation") -> (reference out=w2203:refnum<vi>, error out=w2202:errorcluster)  [unwired: 1 in]
            n1357 = property on="Property Node" class="Bool (strict)"(reference=w2199, "Visible"=FALSE) -> (reference out=w2195:refnum<vi>, error out=w2198:errorcluster)  [unwired: 1 in]
            n1358 = call "DATA ENCRYPT STRING FILE WRITE.vi"("error in (no error)"=w2204, "User Action"="User selected Indentation Mode", "main ref"=w2197) -> ("error out"=w2205:errorcluster)  [unwired: 6 in, 1 out]
            n1359 = Close Reference(reference=w2203, error in (no error)=w2202) -> ()  [unwired: 1 out]
            n1360 = Close Reference(reference=w2195, error in (no error)=w2198) -> ()  [unwired: 1 out]
          }
        }
      }
      frame "SSP 0.3" {
        n1361 = Unbundle By Name(w2209) -> ("Loading.SSP 0.3"=w2212:refnum<vi>)
        n1362 = property on="Property Node" class="Bool (strict)"(reference=w2212, error in=w2211) -> (reference out=w2214:refnum<vi>, error out=w2213:errorcluster, "Value"=w2210:bool)
        n1363 = Close Reference(reference=w2214, error in (no error)=w2213) -> (error out=w2208:errorcluster)
        n1364 = case shown="True" w2210 {
          tunnel: w2209 -> [_ w2216]
          tunnel: w2208 -> [w2215 w2224]
          tunnel: [w2215 w2223] -> w2207
          frame False {
          }
          frame True {
            w2226 = FALSE ("Value")
            n1365 = Unbundle By Name(w2216) -> ("Loading.Enter the Load  (N)"=w2222:refnum<vi>)
            n1366 = Unbundle By Name(w2216) -> ("Loading.SSP 0.75"=w2227:refnum<vi>)
            n1367 = Unbundle By Name(w2216) -> ("Loading.SSP 0.5"=w2232:refnum<vi>)
            n1368 = property on="Property Node" class="Bool (strict)"(reference=w2227, "Value"=w2226) -> (reference out=w2229:refnum<vi>, error out=w2228:errorcluster)  [unwired: 1 in]
            n1369 = property on="Property Node" class="Bool (strict)"(reference=w2232, "Value"=w2226) -> (reference out=w2230:refnum<vi>, error out=w2231:errorcluster)  [unwired: 1 in]
